vi "PI with FF.vi"(0 "Cutoffs":cluster{"MidRange":dbl, "CloseRange":dbl}, 1 "FFcluster":cluster{"FF_m":dbl, "FF_b":dbl}, 2 "ClosePIcluster":cluster{"SlewRate":dbl, "Kp":dbl, "Ki":dbl}, 3 "MidPIcluster":cluster{"SlewRate":dbl, "Kp":dbl, "Ki":dbl}, 4 "FarPIcluster":cluster{"SlewRate":dbl, "Kp":dbl, "Ki":dbl}, 5 "Run PI?":bool, 6 "LimitCluster":cluster{"Step":dbl, "CmdMax":dbl, "CmdMin":dbl}, 7 "SP":dbl, 9 "Actual":dbl, 12 "Freeze Output":bool, 13 "Init (F)":bool) -> (8 "Output":dbl)   [LabVIEW 2013]
uses:
  <vilib>/addons/control/pid/pid.llb/PID Output Rate Limiter (DBL).vi
  <vilib>/addons/control/pid/NI_PID_pid.lvlib
panel:
  in  "2_limit":dbl format="%#_13g"
  in  "2Limit":bool
  out "time":dbl
  in  "Update?":bool
  out "Chart":T1(graph)
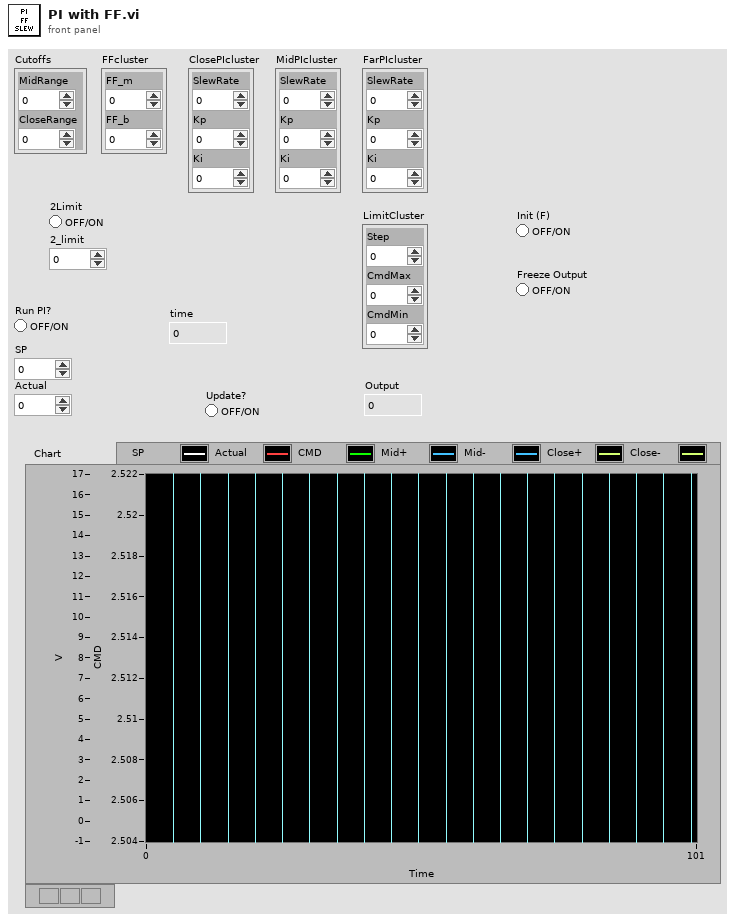
[diagram p1: front panel]
types:
  T1 = cluster{"SP":dbl, "Actual":dbl, dbl, dbl, dbl, dbl, dbl}
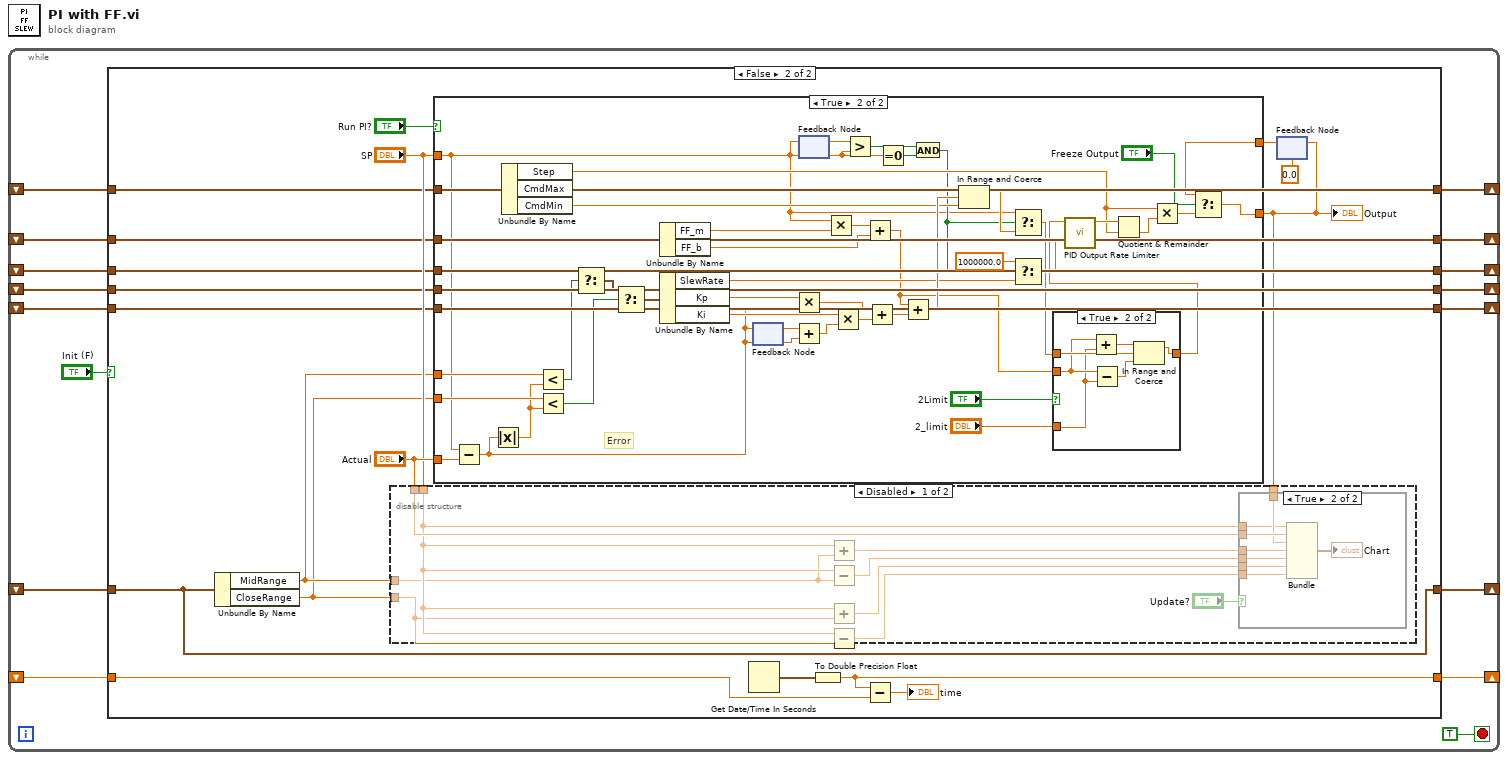
[diagram p0: block diagram]
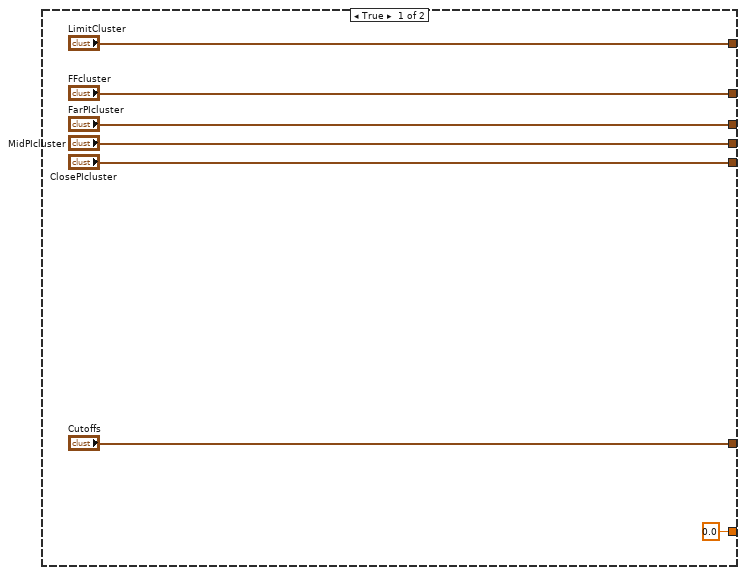
[diagram p2: hidden frame]
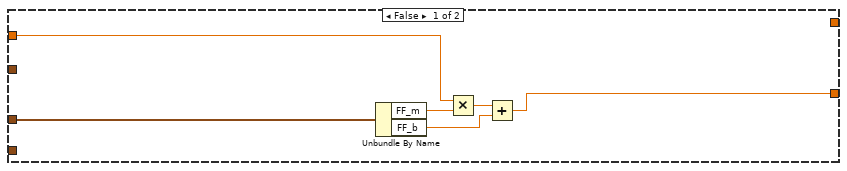
[diagram p5: hidden frame]
diagram:
  n1 = while {
    shift-right: [w14] -> _
    shift-left: _ -> [w13]
    shift-right: [w12] -> _
    shift-left: _ -> [w9]
    shift-right: [w11] -> _
    shift-left: _ -> [w8]
    shift-right: [w10] -> _
    shift-left: _ -> [w7]
    shift-right: [w5] -> _
    shift-left: _ -> [w3]
    shift-right: [w6] -> _
    shift-left: _ -> [w4]
    shift-right: [w2] -> _
    shift-left: _ -> [w1]
    stop <- TRUE stop-if-true
    n2 = case shown="False" "Init (F)" {
      tunnel: ["Cutoffs" w36] -> w14
      tunnel: w13 -> [_ w36]
      tunnel: ["FarPIcluster" w35] -> w12
      tunnel: ["MidPIcluster" w34] -> w11
      tunnel: ["ClosePIcluster" w33] -> w10
      tunnel: w9 -> [_ w35]
      tunnel: w8 -> [_ w34]
      tunnel: w7 -> [_ w33]
      tunnel: ["LimitCluster" w31] -> w6
      tunnel: ["FFcluster" w32] -> w5
      tunnel: w4 -> [_ w31]
      tunnel: w3 -> [_ w32]
      tunnel: [0.0 w28] -> w2
      tunnel: w1 -> [_ w27]
      frame True {
      }
      frame False {
        n3 = Unbundle By Name(w36) -> ("MidRange"=w38:dbl, "CloseRange"=w37:dbl)
        n4 = Get Date/Time In Seconds() -> (seconds since 1Jan1904=w30:timestamp)
        n5 = To Double Precision Float(number=w30) -> (double precision float=w28:dbl)
        n6 = Subtract(x=w28, y=w27) -> (x-y=→"time":dbl)
        n7 = feedback #1(0.0) -> (w26:dbl)
        n8 = case shown="True" "Run PI?" {
          tunnel: [w60 w67] -> w25
          tunnel: "SP" -> [w61 w75]
          tunnel: "Actual" -> [_ w89]
          tunnel: w32 -> [w62 w113]
          tunnel: w35 -> [_ w84]
          tunnel: w31 -> [_ w112]
          tunnel: w34 -> [_ w83]
          tunnel: w33 -> [_ w81]
          tunnel: w38 -> [_ w87]
          tunnel: w37 -> [_ w86]
          tunnel: w26 -> [_ w66]
          frame False {
            n9 = Unbundle By Name(w62) -> ("FF_m"=w64:dbl, "FF_b"=w63:dbl)
            n10 = Multiply(x=w61, y=w64) -> (x*y=w65:dbl)
            n11 = Add(x=w65, y=w63) -> (x+y=w60:dbl)
          }
          frame True {
            # "Error"
            n12 = Subtract(x=w75, y=w89) -> (x-y=w88:dbl)
            n13 = Absolute Value(x=w88) -> (abs(x)=w85:dbl)
            n14 = Unbundle By Name(w112) -> ("Step"=w107:dbl, "CmdMax"=w105:dbl, "CmdMin"=w104:dbl)
            n15 = Less?(x=w87, y=w85) -> (x < y?=w80:bool)
            n16 = Less?(x=w86, y=w85) -> (x < y?=w79:bool)
            n17 = Select(t=w84, s=w80, f=w83) -> (s? t:f=w82:cluster{"SlewRate":dbl, "Kp":dbl, "Ki":dbl})
            n18 = Select(t=w82, s=w79, f=w81) -> (s? t:f=w78:cluster{"SlewRate":dbl, "Kp":dbl, "Ki":dbl})
            n19 = Unbundle By Name(w113) -> ("FF_m"=w97:dbl, "FF_b"=w96:dbl)
            n20 = Unbundle By Name(w78) -> ("SlewRate"=w92:dbl, "Kp"=w111:dbl, "Ki"=w110:dbl)
            n21 = feedback #2(w88) -> (w101:dbl)
            n22 = feedback-in #2(w88) -> ()
            n23 = Multiply(x=w111, y=w88) -> (x*y=w99:dbl)
            n24 = Add(x=w101, y=w88) -> (x+y=w98:dbl)
            n25 = feedback #3(w75) -> (w95:dbl)
            n26 = feedback-in #3(w75) -> ()
            n27 = Multiply(x=w75, y=w97) -> (x*y=w103:dbl)
            n28 = Multiply(x=w110, y=w98) -> (x*y=w100:dbl)
            n29 = Greater?(x=w95, y=w75) -> (0:w94:bool)
            n30 = Add(x=w103, y=w96) -> (x+y=w71:dbl)
            n31 = Add(x=w99, y=w100) -> (x+y=w102:dbl)
            n32 = Equal To 0?(x=w75) -> (x = 0?=w93:bool)
            n33 = Add(x=w71, y=w102) -> (x+y=w106:dbl)
            n34 = And(x=w94, y=w93) -> (x .and. y?=w76:bool)
            n35 = In Range and Coerce(upper limit=w105, x=w106, lower limit=w104) -> (coerced(x)=w77:dbl)  [unwired: 1 out]
            n36 = Select(t=w75, s=w76, f=w77) -> (s? t:f=w73:dbl)
            n37 = Select(t=1000000.0, s=w76, f=w92) -> (s? t:f=w91:dbl)
            n38 = case shown="True" "2Limit" {
              tunnel: w73 -> [w114 w120]
              tunnel: [w114 w119] -> w72
              tunnel: w71 -> [_ w118]
              tunnel: "2_limit" -> [_ w117]
              frame False {
              }
              frame True {
                n39 = Add(x=w118, y=w117) -> (x+y=w115:dbl)
                n40 = Subtract(x=w118, y=w117) -> (x-y=w116:dbl)
                n41 = In Range and Coerce(upper limit=w115, x=w120, lower limit=w116) -> (coerced(x)=w119:dbl)  [unwired: 1 out]
              }
            }
            n42 = call-poly <vilib>:"PID Output Rate Limiter.vi"("output rate (EGU/min)"=w91, "input (controller output)"=w72) -> ("output"=w109:dbl)  [unwired: 6 in, 1 out]
            n43 = Quotient & Remainder(x=w109, y=w107) -> (floor(x/y)=w108:dbl)  [unwired: 1 out]
            n44 = Multiply(x=w107, y=w108) -> (x*y=w68:dbl)
            n45 = Select(t=w66, s="Freeze Output", f=w68) -> (s? t:f=w67:dbl)
          }
        }
        "Output" <- w25
        n46 = disable-structure shown="Disabled" {
          disable-tunnel: "Actual" -> [w51 _]
          disable-tunnel: w25 -> [w50 _]
          disable-tunnel: "SP" -> [w47 _]
          disable-tunnel: w38 -> [w44 _]
          disable-tunnel: w37 -> [w43 _]
          frame Disabled {
            n47 = Add(x=w47, y=w44) -> (x+y=w49:dbl)
            n48 = Subtract(x=w47, y=w44) -> (x-y=w48:dbl)
            n49 = Add(x=w47, y=w43) -> (x+y=w46:dbl)
            n50 = Subtract(x=w47, y=w43) -> (x-y=w45:dbl)
            n51 = case shown="True" "Update?" {
              tunnel: w51 -> [_ w59]
              tunnel: w50 -> [_ w58]
              tunnel: w49 -> [_ w56]
              tunnel: w48 -> [_ w55]
              tunnel: w47 -> [_ w54]
              tunnel: w46 -> [_ w53]
              tunnel: w45 -> [_ w52]
              frame False {
              }
              frame True {
                n52 = Bundle("SP"=w54, "Actual"=w59, w58, w56, w55, w53, w52) -> (→"Chart":T1)  [unwired: 1 in]
              }
            }
          }
          frame Enabled {
          }
        }
        n53 = feedback-in #1(w25) -> ()
      }
    }
  }
